vi "load target runtime.vi"(8 "error in":errorcluster, 11 "target configuration":refnum<class "PL_Target Configuration.lvclass">) -> (0 "error out":errorcluster, 3 "target runtime":refnum<class "PL_Target Runtime.lvclass">)   [LabVIEW 2013, in "PL_Target Runtime.lvclass"]
uses:
  PL_Target Runtime.lvclass
  target configuration/PL_Target Configuration.lvclass
  <vilib>/NI/Tag Bus Module Framework/plugin discovery singleton/class discovery singleton methods.ctl
  <vilib>/NI/Tag Bus Module Framework/plugin discovery singleton/class discovery singleton.lvlib
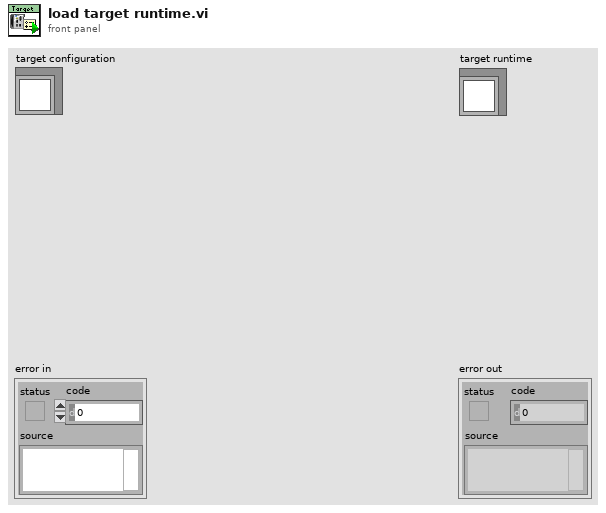
[diagram p1: front panel]
types:
  T1 = typedef "class discovery singleton.lvlib/class discovery singleton methods.ctl" = enum16{"add search paths", "load class by name", "list available classes", "get class path"}
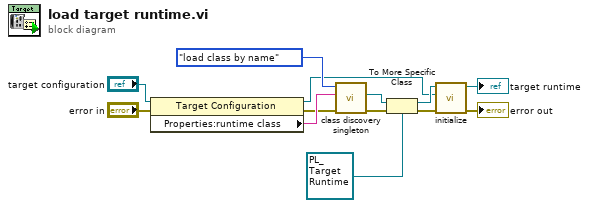
[diagram p0: block diagram]
diagram:
  n1 = property class="Target Configuration"(reference="target configuration", error in="error in") -> (reference out=w1:refnum<class "PL_Target Configuration.lvclass">, error out=w9:errorcluster, "Properties:runtime class"=w11:string)
  n2 = call <vilib>:"class discovery singleton.vi"("error in"=w9, "Class Name"=w11, "method"=class_discovery_singleton_methods."load class by name") -> ("error out"=w8:errorcluster, "LabVIEW Object"=w7:refnum<class>)  [unwired: 5 in, 2 out]
  n3 = To More Specific Class(target class=refnum<class "PL_Target Runtime.lvclass"> refnum ("Target Runtime in"), reference=w7, error in=w8) -> (specific class reference=w3:refnum<class "PL_Target Runtime.lvclass">, error out=w5:errorcluster)
  n4 = call-dynamic "initialize.vi"("error in"=w5, "Target Configuration"=w1, "Target Runtime in"=w3) -> ("error out"=→"error out":errorcluster, "Target Runtime out"=→"target runtime":refnum<class "PL_Target Runtime.lvclass">)  [unwired: 7 in]
